vi "GetMultiInstrumentID.vi"(3 "error in (no error)":errorcluster, 5 "VISA resource name":refnum<visa-resource-name>) -> (0 "error out":errorcluster, 1 "Multi Instrument ID":u8, 2 "VISA resource name out":refnum<visa-resource-name>)   [LabVIEW 2020, in "Active Technologies AWG3000.lvlib"]
uses:
  Active Technologies AWG3000.lvlib
panel:
  out "read buffer":string
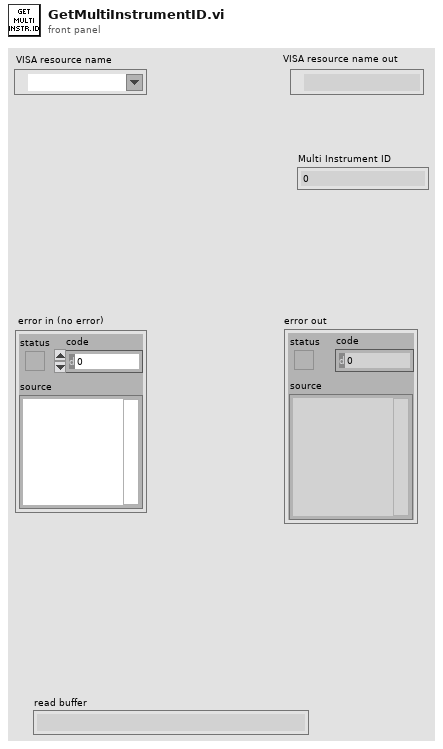
[diagram p1: front panel]
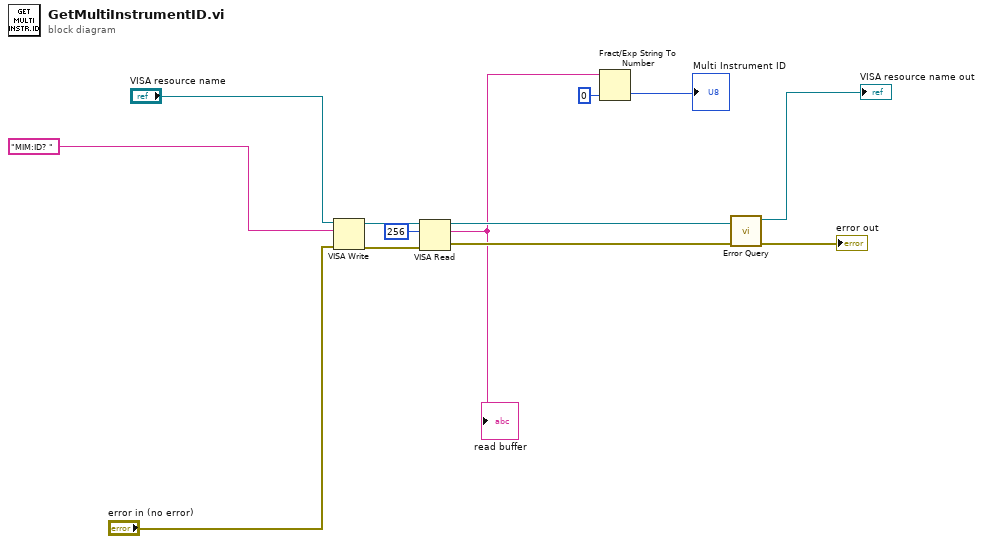
[diagram p0: block diagram]
diagram:
  n1 = VISA Write(VISA resource name="VISA resource name", write buffer="MIM:ID? ", error in (no error)="error in (no error)") -> (VISA resource name out=w11:refnum<visa-resource-name>, error out=w10:errorcluster)  [unwired: 1 out]
  n2 = VISA Read(VISA resource name=w11, byte count=u32 256, error in (no error)=w10) -> (VISA resource name out=w8:refnum<visa-resource-name>, read buffer=w4:string, error out=w7:errorcluster)  [unwired: 1 out]
  "read buffer" <- w4
  n3 = Fract/Exp String To Number(string=w4, default (0 dbl)=u8 0 ("default (0 DBL)")) -> (number=→"Multi Instrument ID":u8)  [unwired: 2 in, 1 out]
  n4 = call "Error Query.vi"("error in (no error)"=w7, "VISA resource name"=w8) -> ("error out"=→"error out":errorcluster, "VISA resource name out"=→"VISA resource name out":refnum<visa-resource-name>)  [unwired: 6 in, 2 out]
